vi "LEDs Streaming.vi"(0 "rx.parameters":T3={"rx.trigger select"=enum."Software", "rx.trigger enable"=FALSE, "rx.trigger sync enable"=FALSE, "rx.stream enable"=[FALSE, FALSE, FALSE, FALSE], "rx.software trigger"=FALSE, "rx.reset"=FALSE, "rx.abort"=FALSE, "rx.samples to acquire"=0, "rx.data sink"=enum."SFP Port 0", "rx.ddc parameters"=[{"output sample rate"=0.0, "delay"=0.0, "frequency shift"=0.0, "impairments"={"inline gain I"=0.0, "inline gain Q"=0.0, "cross gain I"=0.0, "cross gain Q"=0.0, "pre-gain offset I"=0.0, "pre-gain offset Q"=0.0, "post-gain offset I"=0.0, "post-gain offset Q"=0.0}, "phase"=0.0}, {"output sample rate"=0.0, "delay"=0.0, "frequency shift"=0.0, "impairments"={"inline gain I"=0.0, "inline gain Q"=0.0, "cross gain I"=0.0, "cross gain Q"=0.0, "pre-gain offset I"=0.0, "pre-gain offset Q"=0.0, "post-gain offset I"=0.0, "post-gain offset Q"=0.0}, "phase"=0.0}, {"output sample rate"=0.0, "delay"=0.0, "frequency shift"=0.0, "impairments"={"inline gain I"=0.0, "inline gain Q"=0.0, "cross gain I"=0.0, "cross gain Q"=0.0, "pre-gain offset I"=0.0, "pre-gain offset Q"=0.0, "post-gain offset I"=0.0, "post-gain offset Q"=0.0}, "phase"=0.0}, {"output sample rate"=0.0, "delay"=0.0, "frequency shift"=0.0, "impairments"={"inline gain I"=0.0, "inline gain Q"=0.0, "cross gain I"=0.0, "cross gain Q"=0.0, "pre-gain offset I"=0.0, "pre-gain offset Q"=0.0, "post-gain offset I"=0.0, "post-gain offset Q"=0.0}, "phase"=0.0}]} {"rx.ddc parameters"."frequency shift" format="%#.48g"}, 1 "rx.leds":T1, 2 "tx.leds":T2, 5 "rx.status":T8={"rx.state"=enum."Idle", "rx.samples processed"=0, "rx.number of fifo overflows"=0, "rx.number of iq data overflows"=[0, 0], "rx.dsp reset done"=FALSE}, 7 "tx.parameters":T9={"tx.trigger select"=enum."Software", "tx.trigger enable"=FALSE, "tx.trigger sync enable"=FALSE, "tx.stream enable"=[FALSE, FALSE], "tx.software trigger"=FALSE, "tx.reset"=FALSE, "tx.abort"=FALSE, "tx.samples to generate"=0, "tx.data source"=enum."SFP Port 0", "tx.duc parameters"=[{"frequency shift"=0.0, "impairments"={"inline gain I"=0.0, "inline gain Q"=0.0, "cross gain I"=0.0, "cross gain Q"=0.0, "pre-gain offset I"=0.0, "pre-gain offset Q"=0.0, "post-gain offset I"=0.0, "post-gain offset Q"=0.0}, "phase"=0.0, "input sample rate"=0.0, "gain"={"gain I"=0.0, "gain Q"=0.0}, "delay"=0.0}, {"frequency shift"=0.0, "impairments"={"inline gain I"=0.0, "inline gain Q"=0.0, "cross gain I"=0.0, "cross gain Q"=0.0, "pre-gain offset I"=0.0, "pre-gain offset Q"=0.0, "post-gain offset I"=0.0, "post-gain offset Q"=0.0}, "phase"=0.0, "input sample rate"=0.0, "gain"={"gain I"=0.0, "gain Q"=0.0}, "delay"=0.0}]} {"tx.duc parameters"."frequency shift" format="%#.48g"}, 9 "tx.status":T12={"tx.state"=enum."Idle", "tx.samples processed"=0, "tx.number of fifo underflows"=0, "tx.number of iq data overflows"=[0, 0], "tx.dsp reset done"=FALSE}) -> ()   [LabVIEW 2020]
uses:
  Stream Control State.ctl
  Tx Parameters.ctl
  Host/SubVIs/Start Trigger.ctl
  DUC Parameters.ctl
  <instrlib>/_niInstr/DSP/v1/Shared/Public/IQ Impairments.ctl
  <instrlib>/_niInstr/DSP/v1/Shared/Public/IQ Gain.ctl
  Rx Parameters.ctl
  DDC Parameters.ctl
  <instrlib>/_niInstr/Basic Elements/v1/FPGA/Private/Count Down U32.vi
  <vilib>/rvi/eio/common/nirviEmuTemplateMethod_errors.vi
  <vilib>/eio/EIONode/EIONode.xnode
  <instrlib>/_niInstr/Basic Elements/v1/FPGA/niInstr Basic Elements v1 FPGA.lvlib
  <instrlib>/_niInstr/DSP/v1/Shared/niInstr DSP v1 Shared.lvlib
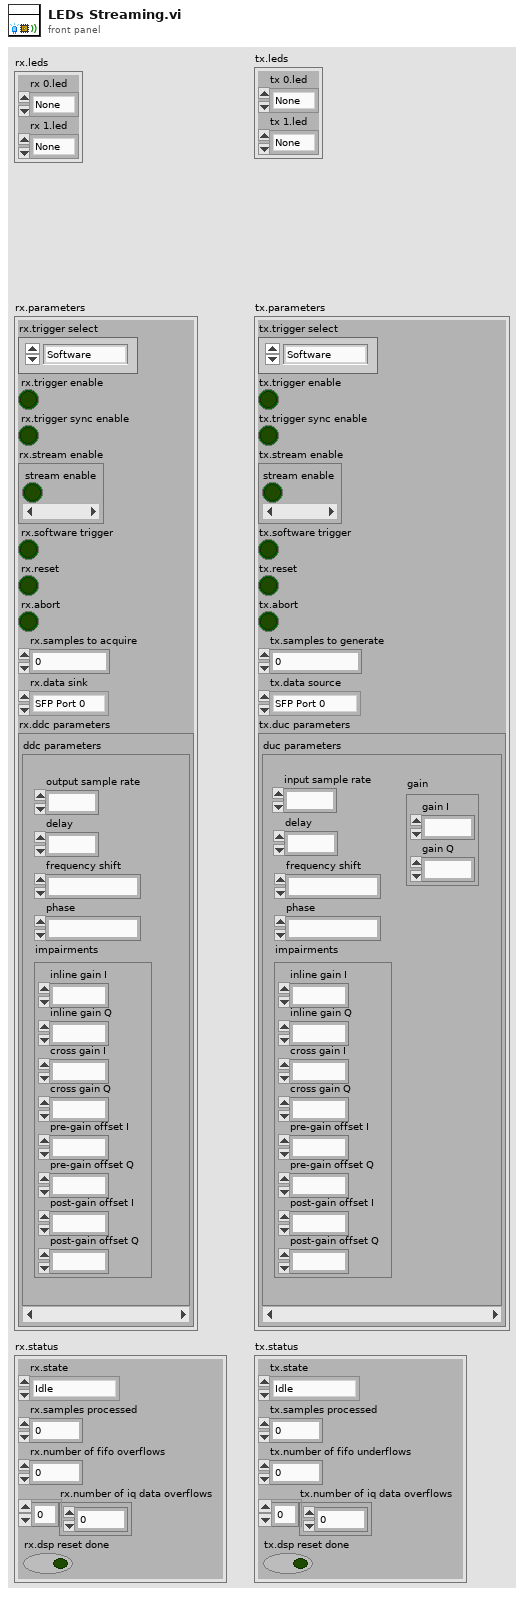
[diagram p1: front panel]
types:
  T1 = cluster{"rx 0.led":enum16{"None", "RF 0/RX 1", "RF 0/RX 2", "RF 1/RX 1", "RF 1/RX 2"}, "rx 1.led":enum16{"None", "RF 0/RX 1", "RF 0/RX 2", "RF 1/RX 1", "RF 1/RX 2"}}
  T2 = cluster{"tx 0.led":enum16{"None", "RF 0/TX 1", "RF 1/TX 1"}, "tx 1.led ":enum16{"None", "RF 0/TX 1", "RF 1/TX 1"}}
  T3 = typedef "Rx Parameters.ctl" = cluster{"rx.trigger select":T4, "rx.trigger enable":bool, "rx.trigger sync enable":bool, "rx.stream enable":bool[], "rx.software trigger":bool, "rx.reset":bool, "rx.abort":bool, "rx.samples to acquire":u32, "rx.data sink":enum16{"SFP Port 0", "SFP Port 1", "Host"}, "rx.ddc parameters":T5[]}
  T4 = typedef "Start Trigger.ctl" = enum8{"Software", "Digital Edge", "Rx Start Trigger", "Tx Start Trigger", "Immediate", "Future Time Event"}
  T5 = typedef "DDC Parameters.ctl" = cluster{"output sample rate":fxp<+,48,1>, "delay":fxp<+/-,16,0>, "frequency shift":fxp<+/-,48,0>, "impairments":T6, "phase":fxp<+/-,21,0>}
  T6 = typedef "niInstr DSP v1 Shared.lvlib/IQ Impairments.ctl" = cluster{"inline gain I":fxp<+/-,18,1>, "inline gain Q":fxp<+/-,18,1>, "cross gain I":fxp<+/-,18,1>, "cross gain Q":fxp<+/-,18,1>, "pre-gain offset I":fxp<+/-,18,1>, "pre-gain offset Q":fxp<+/-,18,1>, "post-gain offset I":fxp<+/-,18,1>, "post-gain offset Q":fxp<+/-,18,1>}
  T7 = typedef "Stream Control State.ctl" = enum16{"Idle", "Active"}
  T8 = cluster{"rx.state":T7, "rx.samples processed":u32, "rx.number of fifo overflows":u32, "rx.number of iq data overflows":u64[], "rx.dsp reset done":bool}
  T9 = typedef "Tx Parameters.ctl" = cluster{"tx.trigger select":T4, "tx.trigger enable":bool, "tx.trigger sync enable":bool, "tx.stream enable":bool[], "tx.software trigger":bool, "tx.reset":bool, "tx.abort":bool, "tx.samples to generate":u32, "tx.data source":enum16{"SFP Port 0", "SFP Port 1", "Host"}, "tx.duc parameters":T10[]}
  T10 = typedef "DUC Parameters.ctl" = cluster{"frequency shift":fxp<+/-,48,0>, "impairments":T6, "phase":fxp<+/-,21,0>, "input sample rate":fxp<+,48,1>, "gain":T11, "delay":fxp<+/-,18,0>}
  T11 = typedef "niInstr DSP v1 Shared.lvlib/IQ Gain.ctl" = cluster{"gain I":fxp<+/-,24,3>, "gain Q":fxp<+/-,24,3>}
  T12 = cluster{"tx.state":T7, "tx.samples processed":u32, "tx.number of fifo underflows":u32, "tx.number of iq data overflows":u64[], "tx.dsp reset done":bool}
  T13 = enum16{"None", "RF 0/RX 1", "RF 0/RX 2", "RF 1/RX 1", "RF 1/RX 2"}
  T14 = enum16{"None", "RF 0/RX 1", "RF 0/RX 2", "RF 1/RX 1", "RF 1/RX 2"}[]
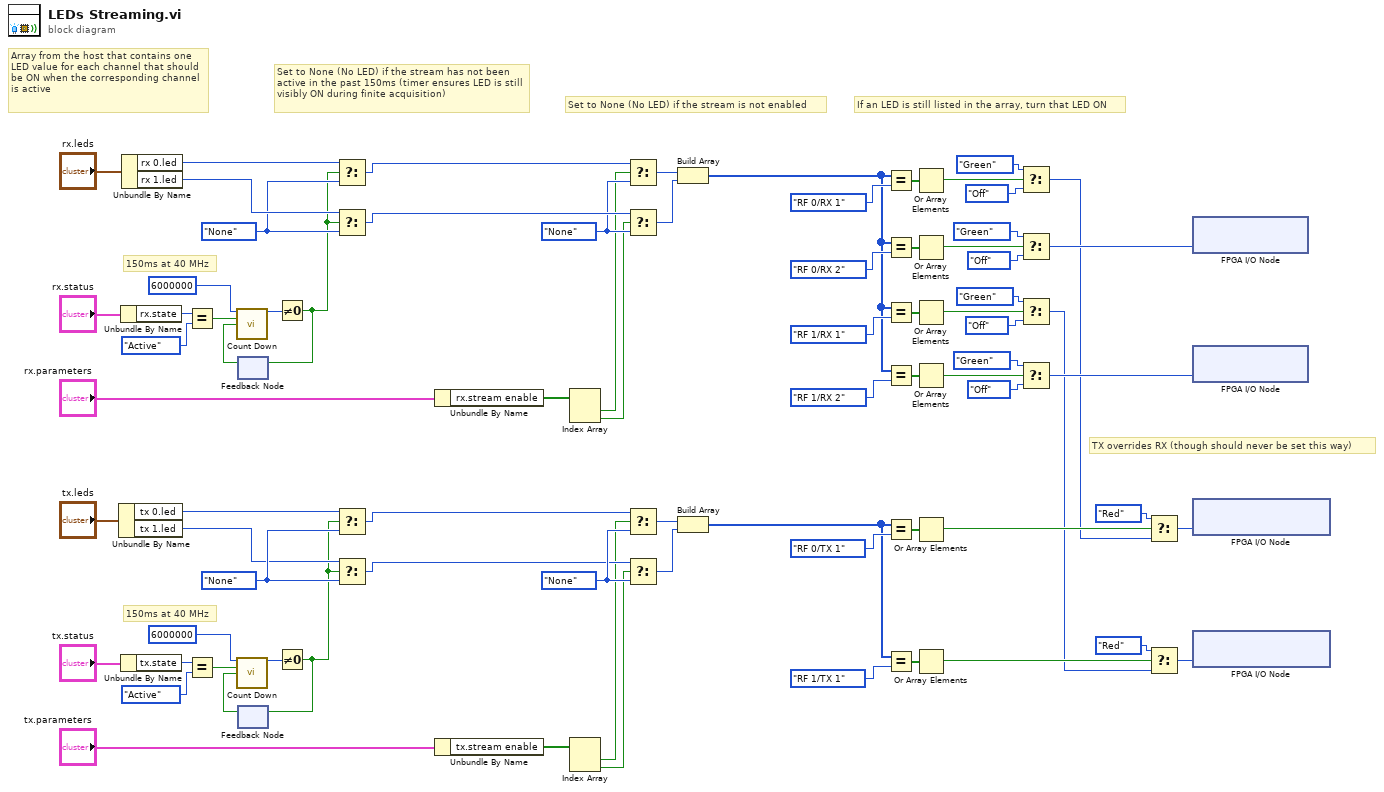
[diagram p0: block diagram]
diagram:
  w31 = enum16{"None", "RF 0/TX 1", "RF 1/TX 1"}."None" ("f")
  w28 = enum16{"None", "RF 0/TX 1", "RF 1/TX 1"}."None" ("f")
  w67 = T13."None" ("f")
  w75 = T13."None" ("f")
  # "TX overrides RX (though should never be set this way)"
  # "If an LED is still listed in the array, turn that LED ON"
  # "Array from the host that contains one LED value for each channel that should be ON when the corresponding channel is active"
  # "Set to None (No LED) if the stream is not enabled"
  # "Set to None (No LED) if the stream has not been active in the past 150ms (timer ensures LED is still visibly ON during finite acquisition)"
  # "150ms at 40 MHz"
  # "150ms at 40 MHz"
  n1 = Unbundle By Name("tx.leds") -> ("tx 0.led"=w26:enum16{"None", "RF 0/TX 1", "RF 1/TX 1"}, "tx 1.led"=w27:enum16{"None", "RF 0/TX 1", "RF 1/TX 1"})
  n2 = Unbundle By Name("rx.status") -> ("rx.state"=w73:T7)
  n3 = Unbundle By Name("tx.status") -> ("tx.state"=w3:T7)
  n4 = Unbundle By Name("rx.leds") -> ("rx 0.led"=w77:T13, "rx 1.led"=w76:T13)
  n5 = Equal?(x=w73, y=Stream_Control_State."Active") -> (x = y?=w13:bool)
  n6 = Equal?(x=w3, y=Stream_Control_State."Active") -> (x = y?=w5:bool)
  n7 = feedback #1() -> (w9:bool)  [unwired: 1 in]
  n8 = call-poly <instrlib>:"Count Down.vi"("count in"=u32 6000000, "load"=w13, "decrement"=w9) -> ("count out"=w11:u32)  [unwired: 11 in, 1 out]
  n9 = feedback #2() -> (w8:bool)  [unwired: 1 in]
  n10 = call-poly <instrlib>:"Count Down.vi"("count in"=u32 6000000, "load"=w5, "decrement"=w8) -> ("count out"=w7:u32)  [unwired: 11 in, 1 out]
  n11 = Not Equal To 0?(x=w11) -> (x != 0?=w10:bool)
  n12 = feedback-in #1(w10) -> ()
  n13 = Not Equal To 0?(x=w7) -> (x != 0?=w1:bool)
  n14 = feedback-in #2(w1) -> ()
  n15 = Select(t=w77, s=w10, f=w75) -> (s? t:f=w69:T13)
  n16 = Select(t=w76, s=w10, f=w75) -> (s? t:f=w68:T13)
  n17 = Select(t=w26, s=w1, f=w28) -> (s? t:f=w29:enum16{"None", "RF 0/TX 1", "RF 1/TX 1"})
  n18 = Select(t=w27, s=w1, f=w28) -> (s? t:f=w30:enum16{"None", "RF 0/TX 1", "RF 1/TX 1"})
  n19 = Unbundle By Name("rx.parameters") -> ("rx.stream enable"=w70:bool[])
  n20 = Unbundle By Name("tx.parameters") -> ("tx.stream enable"=w23:bool[])
  n21 = Index Array(array=w70) -> (element #1=w66:bool, element #2=w65:bool)  [unwired: 2 in]
  n22 = Index Array(array=w23) -> (element #1=w22:bool, element #2=w21:bool)  [unwired: 2 in]
  n23 = Select(t=w69, s=w66, f=w67) -> (s? t:f=w64:T13)
  n24 = Select(t=w68, s=w65, f=w67) -> (s? t:f=w63:T13)
  n25 = Select(t=w29, s=w22, f=w31) -> (s? t:f=w32:enum16{"None", "RF 0/TX 1", "RF 1/TX 1"})
  n26 = Select(t=w30, s=w21, f=w31) -> (s? t:f=w33:enum16{"None", "RF 0/TX 1", "RF 1/TX 1"})
  n27 = Build Array(w64, w63) -> (w47:T14)
  n28 = Build Array(w32, w33) -> (w19:enum16{"None", "RF 0/TX 1", "RF 1/TX 1"}[])
  n29 = Equal?(x=w47, y=T13."RF 0/RX 1" ("f")) -> (x = y?=w61:bool[])
  n30 = Equal?(x=w47, y=T13."RF 0/RX 2" ("f")) -> (x = y?=w56:bool[])
  n31 = Equal?(x=w47, y=T13."RF 1/RX 1" ("f")) -> (x = y?=w53:bool[])
  n32 = Equal?(x=w47, y=T13."RF 1/RX 2" ("f")) -> (x = y?=w49:bool[])
  n33 = Equal?(x=w19, y=enum16{"None", "RF 0/TX 1", "RF 1/TX 1"}."RF 0/TX 1" ("f")) -> (x = y?=w34:bool[])
  n34 = Equal?(x=w19, y=enum16{"None", "RF 0/TX 1", "RF 1/TX 1"}."RF 1/TX 1" ("f")) -> (x = y?=w37:bool[])
  n35 = Or Array Elements(Boolean array=w61) -> (logical OR=w60:bool)
  n36 = Or Array Elements(Boolean array=w56) -> (logical OR=w57:bool)
  n37 = Or Array Elements(Boolean array=w53) -> (logical OR=w52:bool)
  n38 = Or Array Elements(Boolean array=w49) -> (logical OR=w41:bool)
  n39 = Or Array Elements(Boolean array=w34) -> (logical OR=w35:bool)
  n40 = Or Array Elements(Boolean array=w37) -> (logical OR=w38:bool)
  n41 = Select(t=enum8{"Off", "Green", "Red", "Amber"}."Green" ("LED/RF 0/TX1 RX1"), s=w60, f=enum8{"Off", "Green", "Red", "Amber"}."Off" ("LED/RF 0/TX1 RX1")) -> (s? t:f=w17:enum8{"Off", "Green", "Red", "Amber"})
  n42 = Select(t=enum8{"Off", "Green"}."Green" ("LED/RF 0/RX2"), s=w57, f=enum8{"Off", "Green"}."Off" ("LED/RF 0/RX2")) -> (s? t:f=w44:enum8{"Off", "Green"})
  n43 = Select(t=enum8{"Off", "Green", "Red", "Amber"}."Green" ("LED/RF 0/TX1 RX1"), s=w52, f=enum8{"Off", "Green", "Red", "Amber"}."Off" ("LED/RF 0/TX1 RX1")) -> (s? t:f=w15:enum8{"Off", "Green", "Red", "Amber"})
  n44 = Select(t=enum8{"Off", "Green"}."Green" ("LED/RF 0/RX2"), s=w41, f=enum8{"Off", "Green"}."Off" ("LED/RF 0/RX2")) -> (s? t:f=w40:enum8{"Off", "Green"})
  n45 = Select(t=enum8{"Off", "Green", "Red", "Amber"}."Red" ("LED/RF 0/TX1 RX1"), s=w35, f=w17) -> (s? t:f=w16:enum8{"Off", "Green", "Red", "Amber"})
  n46 = Select(t=enum8{"Off", "Green", "Red", "Amber"}."Red" ("LED/RF 0/TX1 RX1"), s=w38, f=w15) -> (s? t:f=w14:enum8{"Off", "Green", "Red", "Amber"})
  n47 = xnode "FPGA I/O Node"("LED/RF 0/RX2"=w44) -> ()  [unwired: 1 in, 1 out]
  n48 = xnode "FPGA I/O Node"("LED/RF 1/RX2"=w40) -> ()  [unwired: 1 in, 1 out]
  n49 = xnode "FPGA I/O Node"("LED/RF 0/TX1 RX1"=w16) -> ()  [unwired: 1 in, 1 out]
  n50 = xnode "FPGA I/O Node"("LED/RF 1/TX1 RX1"=w14) -> ()  [unwired: 1 in, 1 out]
